vi "海流计数据组合.vi"(10 "不再发送":bool, 11 "要发送的海流计参数":string[][](array[string])) -> (3 "发送的信息":string)   [LabVIEW 2016, in "数据传输系统-04.lvlib"]
panel:
  out "层数参数位置":i32
  out "层数":string
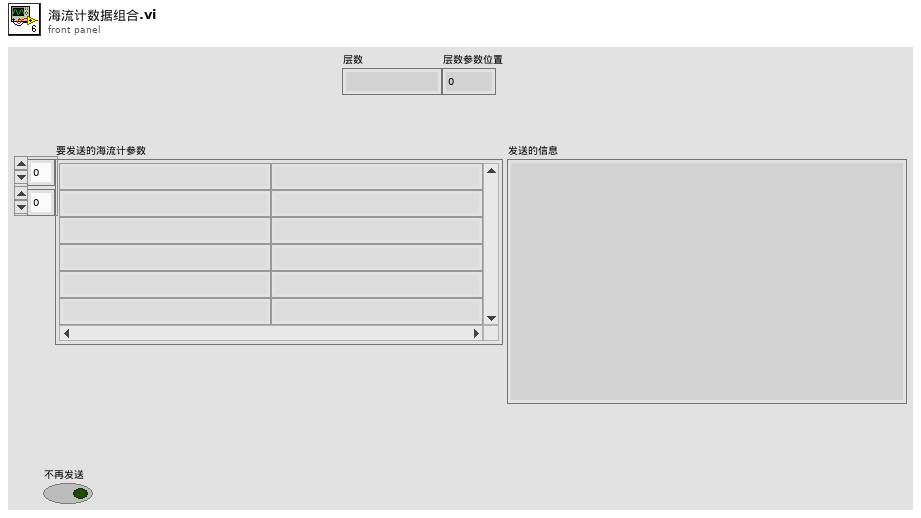
[diagram p1: front panel]
types:
  T1 = cluster{"CODMn":string, "CODCr":string, "DO":string, "铜":string, "PH":string, "氨氮":string, "比电导率":string, "水温":string, "COD":string, "浊度":string, "总氮":string, "总磷":string, "叶绿素a":string, "藻密度":string, "水位":string, "流速":string, "方向":string, "瞬时流量":string, "累积流量":string, "正累积流量":string, "负累积流量":string, "亚硝酸盐":string, "硫化物":string, "ORP":string, "铅":string, "镉":string, "锌":string, "镍":string, "锰":string, "汞":string, "气温":string, "气压":string, "风速":string, "风向":string, "空气温度":string, "相对湿度":string, "分钟雨量":string, "小时雨量":string, "日雨量":string, "累积雨量":string, "盐度":string, "磷酸盐":string, "硝氮":string, "氟化物":string, "挥发酚":string, "氯化物":string, "蓝绿藻":string, "余氯":string, "综合生物毒性":string, "艏向":string, "横摇":string, "纵摇":string, "分层标志":string, "层状态1":string, "层状态2":string, "水平平均流速":string, "流向":string, "北向流速分量":string, "东向流速分量":string, "垂直流速分量":string, "最大波高":string, "最大波周期":string, "1/10波高":string, "1/10波周期":string, "有效波高":string, "有效波周期":string, "平均波高":string, "平均波周期":string, "波向":string, "波个数":string, "水深":string, "X轴流速":string, "Y轴流速":string, "信号强度":string, "电压":string, "悬浮物":string}
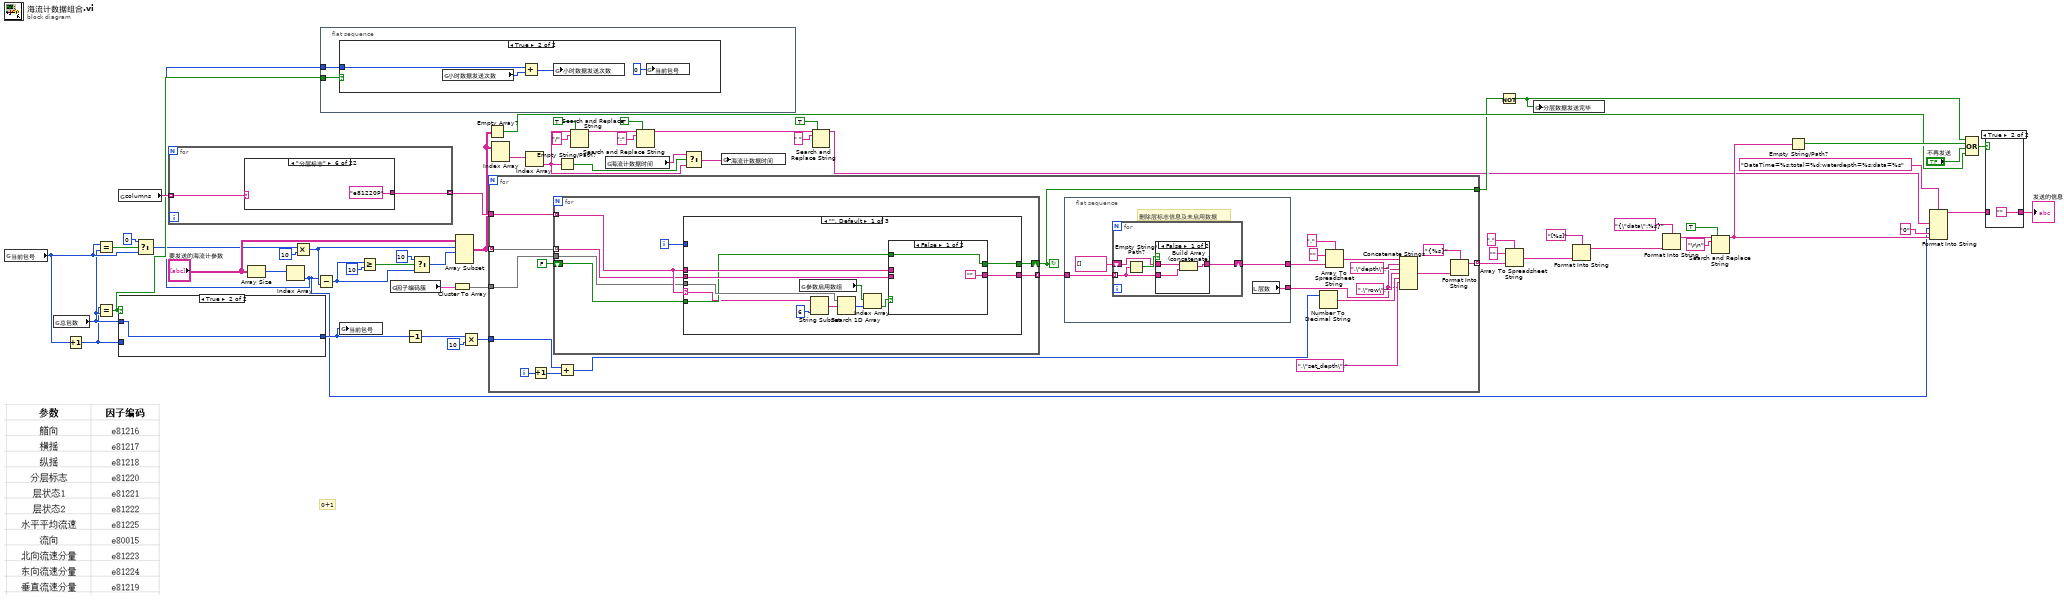
[diagram p0: block diagram]
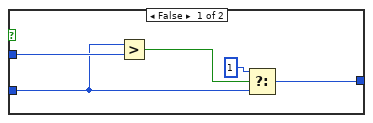
[diagram p2: hidden frame]
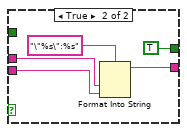
[diagram p6: hidden frame]
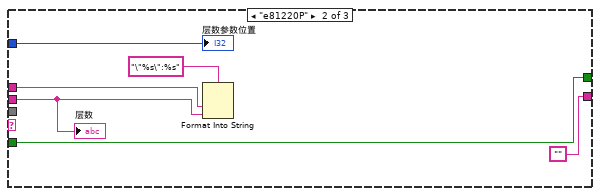
[diagram p7: hidden frame]
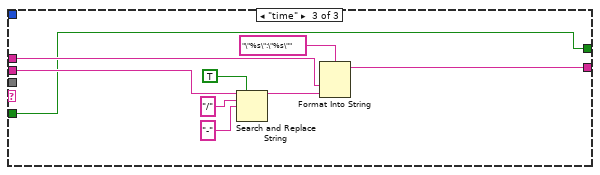
[diagram p8: hidden frame]
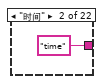
[diagram p10: hidden frame]
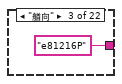
[diagram p11: hidden frame]
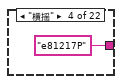
[diagram p12: hidden frame]
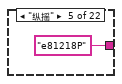
[diagram p13: hidden frame]
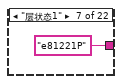
[diagram p14: hidden frame]
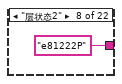
[diagram p15: hidden frame]
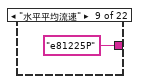
[diagram p16: hidden frame]
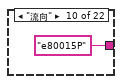
[diagram p17: hidden frame]
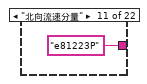
[diagram p18: hidden frame]
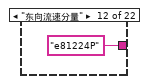
[diagram p19: hidden frame]
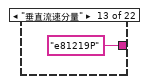
[diagram p20: hidden frame]
diagram:
  # "0+1"
  n1 = global read "全局 数据数组大小.vi" "当前包号"() -> (w30:i32)
  n2 = global read "全局 数据数组大小.vi" "总包数"() -> (w27:i32)
  n3 = Increment(x=w30) -> (x+1=w1:i32)
  n4 = Equal?(x=w30, y=w27) -> (x = y?=w31:bool)
  n5 = Equal?(x=w1, y=w27) -> (x = y?=w32:bool)
  n6 = global read "全局 所有参数.vi" "columns"() -> (w47:string[])
  n7 = case shown="True" w32 {
    tunnel: [w65 w67] -> w26
    tunnel: w1 -> [w62 _]
    tunnel: w27 -> [w66 w67]
    frame False {
      n8 = Greater?(x=w62, y=w66) -> (0:w64:bool)
      n9 = Select(t=1, s=w64, f=w62) -> (s? t:f=w65:i32)
    }
    frame True {
    }
  }
  n10 = Select(t=0, s=w31, f=w30) -> (s? t:f=w28:i32)
  n11 = for {
    tunnel: w47 -> [w69] mode=indexing
    tunnel: [w68] -> w51 mode=indexing
    n12 = case shown="\"分层标志\"" w69 {
      tunnel: [_ "time" ("元素") "e81216P" "e81217P" "e81218P" "e81220P" "e81221P" "e81222P" "e81225P" "e80015P" "e81223P" "e81224P" "e81219P" "w00004P" "w00005P" "w00006P" "w00007P" "w01002P" "w01022P" "w81024P" "w81025P" "w81023P"] -> w68
      frame "", Default {
      }
      frame "时间" {
      }
      frame "艏向" {
      }
      frame "横摇" {
      }
      frame "纵摇" {
      }
      frame "分层标志" {
      }
      frame "层状态1" {
      }
      frame "层状态2" {
      }
      frame "水平平均流速" {
      }
      frame "流向" {
      }
      frame "北向流速分量" {
      }
      frame "东向流速分量" {
      }
      frame "垂直流速分量" {
      }
      frame "隐藻" {
      }
      frame "透光率" {
      }
      frame "黄色物质" {
      }
      frame "总藻" {
      }
      frame "盐度" {
      }
      frame "蓝绿藻" {
      }
      frame "Fv/Fm" {
      }
      frame "PAR" {
      }
      frame "GPP" {
      }
    }
  }
  n13 = Array Size(array="要发送的海流计参数") -> (size(s)=w40:i32[])
  n14 = Index Array(array=w40) -> (element=w3:i32)  [unwired: 1 in]
  n15 = Multiply(x=w28, y=10) -> (x*y=w33:i32)
  n16 = Subtract(x=w3, y=w33) -> (x-y=w35:i32)
  n17 = flat-sequence {
    tunnel: w32 -> [w92]
    tunnel: w3 -> [w91]
    frame #0 {
      n18 = case shown="True" w92 {
        tunnel: w91 -> [_ w96]
        frame False {
        }
        frame True {
          n19 = global read "全局 小时数据发送次数.vi" "小时数据发送次数"() -> (w95:i32)
          n20 = Add(x=w96, y=w95) -> (x+y=w94:i32)
          n21 = global write "全局 小时数据发送次数.vi" "小时数据发送次数"(w94) -> ()
          n22 = global write "全局 数据数组大小.vi" "当前包号"(0 ("当前包号")) -> ()
        }
      }
    }
  }
  n23 = global write "全局 数据数组大小.vi" "当前包号"(w26) -> ()
  n24 = Greater Or Equal?(x=w35, y=10) -> (x >= y?=w37:bool)
  n25 = global read "断电保存全局.vi" "因子编码簇"() -> (w7:T1)
  n26 = Decrement(x=w26) -> (x-1=w25:i32)
  n27 = Select(t=10 ("y"), s=w37, f=w35) -> (s? t:f=w34:i32)
  n28 = Cluster To Array(cluster=w7) -> (array=w6:string[])
  n29 = Array Subset(array="要发送的海流计参数", index (row)=w33, length (row)=w34) -> (w20:string[][])  [unwired: 2 in]
  n30 = Multiply(x=w25, y=10) -> (x*y=w23:i32)
  n31 = Empty Array?(array=w20) -> (empty?=w22:bool)
  n32 = for {
    tunnel: w20 -> [w117] mode=indexing
    tunnel: w51 -> [w118]
    tunnel: [w113] -> w59 mode=indexing
    tunnel: w23 -> [w103]
    tunnel: w6 -> [w99]
    tunnel: [w97] -> w5
    i -> [w112]
    stop <- w97 continue-if-true
    n33 = Increment(x=w112) -> (x+1=w104:i32)
    n34 = for {
      tunnel: w118 -> [w136] mode=indexing
      tunnel: w117 -> [w135] mode=indexing
      tunnel: [w137] -> w102 mode=indexing
      tunnel: w99 -> [w133]
      shift-right: [w131] -> w97
      shift-left: FALSE -> [w132]
      i -> [w134]
      n35 = case shown="\"\", Default" w136 {
        selector: w136 -> [w141 _ _]
        tunnel: [w149 "" w170] -> w137
        tunnel: w136 -> [w148 w161 w169]
        tunnel: w135 -> [w147 w160 w165]
        tunnel: w134 -> [_ w159 _]
        tunnel: w133 -> [w146 _ _]
        tunnel: w132 -> [w142 w157 w163]
        tunnel: [w143 w157 w163] -> w131
        frame "", Default {
          n36 = global read "断电保存全局.vi" "参数启用数组"() -> (w145:bool[])
          n37 = String Subset(string=w141, length (rest)=6 ("长度（剩余）")) -> (substring=w139:string)  [unwired: 1 in]
          n38 = Search 1D Array(1D array=w146, element=w139) -> (index of element=w144:i32)  [unwired: 1 in]
          n39 = Index Array(array=w145, index=w144) -> (element=w138:bool)
          n40 = case shown="False" w138 {
            tunnel: ["" w155] -> w149
            tunnel: w148 -> [_ w154]
            tunnel: w147 -> [_ w153]
            tunnel: [w150 TRUE] -> w143
            tunnel: w142 -> [w150 _]
            frame False {
            }
            frame True {
              n41 = Format Into String(format string="\"%s\":%s" ("格式字符串"), w154, w153) -> (resulting string=w155:string)  [unwired: 2 in, 1 out]
            }
          }
        }
        frame "e81220P" {
          n42 = Format Into String(format string="\"%s\":%s" ("格式字符串"), w161, w160) -> ()  [unwired: 2 in, 2 out]
          "层数" <- w160
          "层数参数位置" <- w159
        }
        frame "time" {
          n43 = Search and Replace String(replace all?=TRUE ("替换全部？(F)"), input string=w165, search string="/" ("搜索字符串"), replace string="-" ("替换字符串(\"\")")) -> (result string=w164:string)  [unwired: 4 in, 3 out]
          n44 = Format Into String(format string="\"%s\":\"%s\"" ("格式字符串"), w169, w164) -> (resulting string=w170:string)  [unwired: 2 in, 1 out]
        }
      }
    }
    n45 = Add(x=w103, y=w104) -> (x+y=w105:i32)
    n46 = flat-sequence {
      tunnel: w102 -> [w121]
      tunnel: [w122] -> w101
      tunnel: [w119] -> w100
      frame #0 {
        # "删除层标志信息及未启用数据"
        n47 = for {
          tunnel: w121 -> [w123] mode=indexing
          shift-right: [w124] -> w119
          shift-left: string[] [] -> [w125]
          n48 = Empty String/Path?(string/path=w123) -> (empty?=w126:bool)
          n49 = case shown="False" w126 {
            tunnel: [w127 w130] -> w124
            tunnel: w125 -> [w129 w130]
            tunnel: w123 -> [w128 _]
            frame False {
              n50 = Build Array (concatenate)(w129, w128) -> (w127:string[])
            }
            frame True {
            }
          }
        }
        n51 = local read "层数"() -> (w122:string)
      }
    }
    n52 = Number To Decimal String(number=w105) -> (decimal integer string=w109:string)  [unwired: 1 in]
    n53 = Array To Spreadsheet String(delimiter (Tab)="," ("分隔符(Tab)"), array=w100, 3:"" ("格式字符串")) -> (spreadsheet string=w107:string)
    n54 = Concatenate Strings(w107, ",\"depth\":", w101, ",\"row\":", w109, ",\"set_depth\":", w101) -> (w106:string)
    n55 = Format Into String(format string="{%s}" ("格式字符串"), w106) -> (resulting string=w113:string)  [unwired: 2 in, 1 out]
  }
  n56 = Index Array(array=w20) -> (element=w21:string[])  [unwired: 2 in]
  n57 = Index Array(array=w21) -> (element=w10:string)  [unwired: 1 in]
  n58 = Empty String/Path?(string/path=w10) -> (empty?=w11:bool)
  n59 = Search and Replace String(replace all?=TRUE ("替换全部？(F)"), input string=w10, search string="/" ("替换字符串(\"\")")) -> (result string=w15:string)  [unwired: 5 in, 3 out]
  n60 = global read "全局 水样时间.vi" "海流计数据时间"() -> (w9:string)
  n61 = Search and Replace String(replace all?=TRUE ("替换全部？(F)"), input string=w15, search string=":" ("替换字符串(\"\")")) -> (result string=w12:string)  [unwired: 5 in, 3 out]
  n62 = Select(t=w9, s=w11, f=w10) -> (s? t:f=w8:string)
  n63 = global write "全局 水样时间.vi" "海流计数据时间"(w8) -> ()
  n64 = Search and Replace String(replace all?=TRUE ("替换全部？(F)"), input string=w12, search string=" " ("替换字符串(\"\")")) -> (result string=w2:string)  [unwired: 5 in, 3 out]
  n65 = Not(x=w5) -> (.not. x?=w4:bool)
  n66 = Array To Spreadsheet String(delimiter (Tab)="," ("分隔符(Tab)"), array=w59, 3:"" ("格式字符串")) -> (spreadsheet string=w55:string)
  n67 = global write "全局 数据数组大小.vi" "分层数据发送完毕"(w4) -> ()
  n68 = Format Into String(format string="[%s]" ("格式字符串"), w55) -> (resulting string=w56:string)  [unwired: 2 in, 1 out]
  n69 = Format Into String(format string="{\"data\":%s}" ("格式字符串"), w56) -> (resulting string=w52:string)  [unwired: 2 in, 1 out]
  n70 = Search and Replace String(replace all?=TRUE ("替换全部？(F)"), input string=w52, search string="\r\n") -> (result string=w46:string)  [unwired: 5 in, 3 out]
  n71 = Empty String/Path?(string/path=w46) -> (empty?=w44:bool)
  n72 = Format Into String(format string="DataTime=%s;total=%d;waterdepth=%s;data=%s", w2, w3, "0" ("输入 3"), w46) -> (resulting string=w49:string)  [unwired: 2 in, 1 out]
  n73 = Compound Arithmetic op=OR ("复合运算")(w4, w44, "不再发送", w22) -> (w42:bool)
  n74 = case shown="True" w42 {
    tunnel: [w172 ""] -> w48
    tunnel: w49 -> [w172 _]
    frame False {
    }
    frame True {
    }
  }
  "发送的信息" <- w48
